vi "pendiente_recta.vi"() -> ()   [LabVIEW 2020]
panel:
  in  "stop":bool
  out "Cruce x Cero (b)":dbl
  out "Pendiente":dbl
  in  "x1":dbl
  in  "x2":dbl
  in  "y1":dbl
  in  "y2":dbl
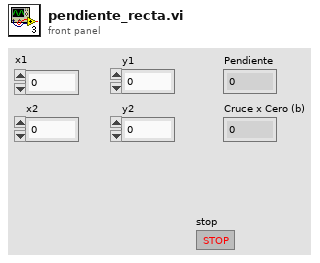
[diagram p1: front panel]
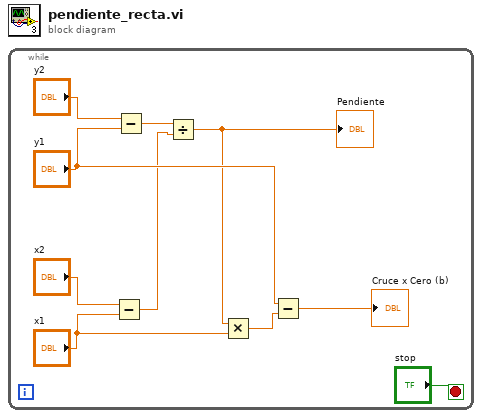
[diagram p0: block diagram]
diagram:
  n1 = while {
    stop <- "stop" stop-if-true
    n2 = Subtract(x="x2", y="x1") -> (x-y=w4:dbl)
    n3 = Subtract(x="y2", y="y1") -> (x-y=w9:dbl)
    n4 = Divide(x=w9, y=w4) -> (x/y=w2:dbl)
    "Pendiente" <- w2
    n5 = Multiply(x=w2, y="x1") -> (x*y=w6:dbl)
    n6 = Subtract(x="y1", y=w6) -> (x-y=→"Cruce x Cero (b)":dbl)
  }
